vi "VI Tree.vi"   [LabVIEW 2013, in "HadCon.lvlib"]
doc: "This is the instrument driver for the <INSTRUMENT NAME>. The VI Tree displays all the user-callable VIs of the instrument driver in an organized table."
uses:
  <instrlib>/HadCon/HadCon.lvlib
panel:
  # "(c) 2014 GSI Helmholtzzentrum für Schwerionenforschung GmbH.  ALL RIGHTS RESERVED.\nLizenziert unter EUPL V. 1.1"
  # "SEE DIAGRAM\nFOR VI TREE."
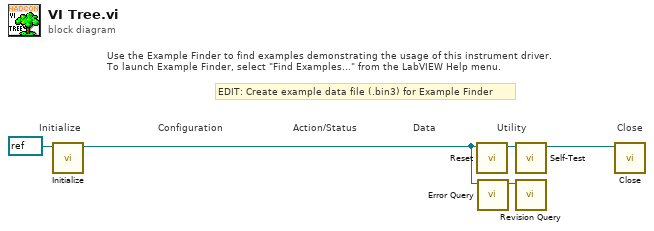
[diagram p0: block diagram]
diagram:
  # "EDIT: Create example data file (.bin3) for Example Finder"
  # "Use the Example Finder to find examples demonstrating the usage of this instrument driver.\nTo launch Example Finder, select \"Find Examples...\" from the LabVIEW Help menu."
  # "Configuration"
  # "Utility"
  # "Data"
  # "Action/Status"
  # "Close"
  # "Initialize"
  n1 = call <instrlib>:"Initialize.vi"("VISA resource name"=refnum<visa-resource-name> refnum) -> ("VISA resource name out"=w4:refnum<visa-resource-name>)  [unwired: 9 in, 1 out]
  n2 = call <instrlib>:"Reset.vi"("VISA resource name"=w4) -> ("VISA resource name out"=w3:refnum<visa-resource-name>)  [unwired: 9 in, 1 out]
  n3 = call <instrlib>:"Error Query.vi"("VISA resource name"=w4) -> ("VISA resource name out"=w2:refnum<visa-resource-name>)  [unwired: 7 in, 3 out]
  n4 = call <instrlib>:"Self-Test.vi"("VISA resource name"=w3) -> ("VISA resource name out"=w1:refnum<visa-resource-name>)  [unwired: 7 in, 3 out]
  n5 = call <instrlib>:"Revision Query.vi"("VISA resource name"=w2) -> ()  [unwired: 7 in, 4 out]
  n6 = call <instrlib>:"Close.vi"("VISA resource name"=w1) -> ()  [unwired: 10 in, 1 out]
